vi "FGVtable.vi"(8 "error in":errorcluster, 10 "Write from FGV or Read from FGV?":T1, 11 "Input Value":bool=TRUE) -> (0 "error out":errorcluster, 3 "Output Value":bool)   [LabVIEW 2014]
uses:
  Controls/FGVisfileopen.ctl
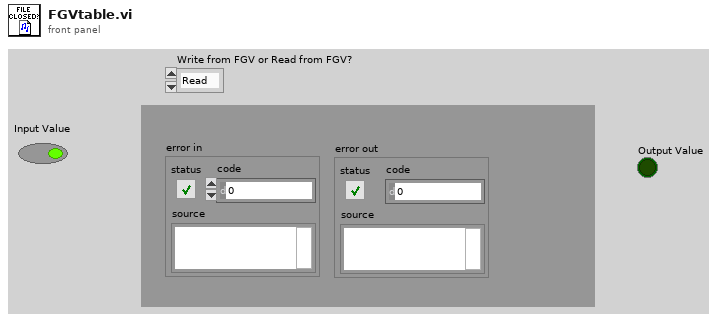
[diagram p1: front panel]
types:
  T1 = typedef "FGVisfileopen.ctl" = enum16{"Read", "Write"}
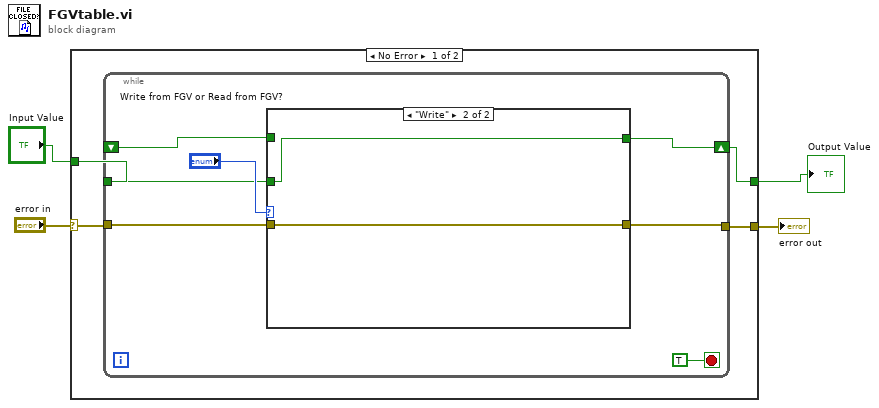
[diagram p0: block diagram]
diagram:
  n1 = case shown="No Error" "error in" {
    selector: "error in" -> [w7 w21]
    tunnel: [w8 w21] -> w4
    tunnel: "Input Value" -> [w6 w20]
    tunnel: [w5 w20] -> w2
    frame No Error {
      n2 = while {
        tunnel: w7 -> [w10]
        tunnel: [w9] -> w8
        tunnel: w6 -> [w13]
        shift-right: [w12] -> w5
        shift-left: _ -> [w11]
        stop <- TRUE stop-if-true
        n3 = case shown="\"Write\"" "Write from FGV or Read from FGV?" {
          tunnel: w13 -> [_ w18]
          tunnel: [w16 w18] -> w12
          tunnel: w11 -> [w16 _]
          tunnel: [w17 w19] -> w9
          tunnel: w10 -> [w17 w19]
          frame "Read", Default {
          }
          frame "Write" {
          }
        }
      }
    }
    frame Error {
    }
  }
  "error out" <- w4
  "Output Value" <- w2
